vi "Check If Value Is In Range.vi"(9 "Value":dbl, 11 "Range String":string) -> (1 "In Range?":bool, 2 "Lower":dbl, 3 "Upper":dbl)   [LabVIEW 2025, in "Test Limits.lvlib"]
uses:
  Test Limits.lvlib
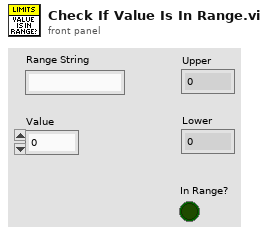
[diagram p1: front panel]
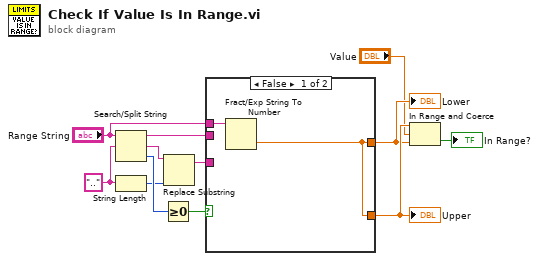
[diagram p0: block diagram]
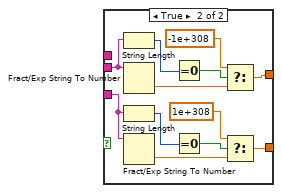
[diagram p2: hidden frame]
diagram:
  w12 = ".." ("search string/char (-)")
  n1 = Search/Split String(string="Range String", search string/char (-)=w12) -> (substring before match=w10:string, match + rest of string=w6:string, offset of match=w11:i32)  [unwired: 1 in]
  n2 = String Length(string=w12) -> (length=w7:i32)
  n3 = Greater Or Equal To 0?(x=w11) -> (x >= 0?=w9:bool)
  n4 = Replace Substring(2:w7, 5:w6) -> (1:w5:string)  [unwired: 2 in, 1 out]
  n5 = case shown="False" w9 {
    tunnel: [w13 w23] -> w4
    tunnel: [w13 w19] -> w3
    tunnel: w10 -> [_ w18]
    tunnel: "Range String" -> [w14 _]
    tunnel: w5 -> [_ w15]
    frame False {
      n6 = Fract/Exp String To Number(string=w14) -> (number=w13:dbl)  [unwired: 3 in, 1 out]
    }
    frame True {
      n7 = String Length(string=w18) -> (length=w21:i32)
      n8 = Fract/Exp String To Number(string=w18) -> (number=w17:dbl)  [unwired: 3 in, 1 out]
      n9 = String Length(string=w15) -> (length=w26:i32)
      n10 = Fract/Exp String To Number(string=w15) -> (number=w24:dbl)  [unwired: 3 in, 1 out]
      n11 = Equal To 0?(x=w21) -> (x = 0?=w20:bool)
      n12 = Equal To 0?(x=w26) -> (x = 0?=w25:bool)
      n13 = Select(t=-1e+308, s=w20, f=w17) -> (s? t:f=w19:dbl)
      n14 = Select(t=1e+308, s=w25, f=w24) -> (s? t:f=w23:dbl)
    }
  }
  "Upper" <- w4
  "Lower" <- w3
  n15 = In Range and Coerce(upper limit=w4, x="Value", lower limit=w3) -> (In Range?=→"In Range?":bool)  [unwired: 1 out]
